vi "Initialize Steps Tree.vi"(11 "UI Data in":refnum<class "Settings UI.lvclass">) -> (2 "Items to Add":T1(array[cluster]), 3 "UI Data out":refnum<class "Settings UI.lvclass">)   [LabVIEW 2020, in "Output Sequencer.lvlib" / "Settings UI.lvclass"]
uses:
  Settings UI.lvclass
  Types/Tree Index Enum.ctl
  Settings UI.lvclass/Settings UI.ctl
  Globals/Global Tree Data.vi
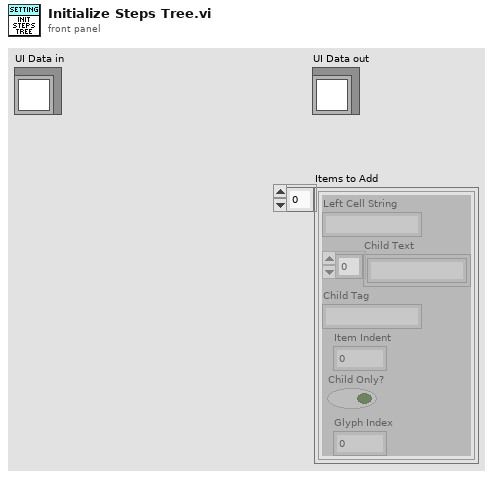
[diagram p1: front panel]
types:
  T1 = cluster{"Left Cell String":string, "Child Text":string[], "Child Tag":string, "Item Indent":i32, "Child Only?":bool, "Glyph Index":i32}[]
  T2 = typedef "Output Sequencer.lvlib/Settings UI.lvclass/Tree Index Enum.ctl" = enum16{"General Settings", "Num Steps", "Num Analog", "Num Digital", "Show Confirmation", "Interp Priority", "Adv Timing", "Enable Conditions", "Seq Execution", "Reset Test Start", "Only When Test", "Delay After Test", "Start condition", "Re-triggering", "Stop condition", "Stop After Cycles", "Stop Values", "Default Values", "Default Analog", "Default Digital", "Steps", "Step #", "Description", "Precondition", "Duration", "Mode", "Delay Between Vals", "Analog Values", "Digital Values", "Postcondition", "On True", "On False"}
  T3 = typedef "Output Sequencer.lvlib/Settings UI.lvclass/Step Settings.ctl" = cluster{"Description":string, "Precondition":string, "Duration":dbl, "Mode":string, "Delay Between Values":dbl, "Analog Values":string[], "Digital Values":string[], "Postcondition":string, "On True":string, "On False":string}
  T4 = cluster{"Left Cell String":string, "Child Text":string[], "Child Tag":string, "Item Indent":i32, "Child Only?":bool, "Glyph Index":i32}
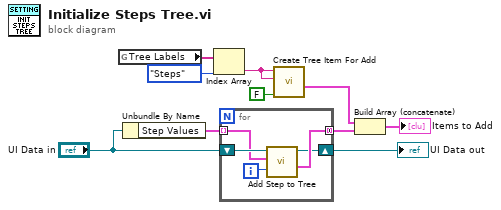
[diagram p0: block diagram]
diagram:
  n1 = global read "Global Tree Data.vi" "Tree Labels"() -> (w7:string[])
  n2 = Unbundle By Name("UI Data in") -> ("Step Values"=w8:T3[])
  n3 = Index Array(array=w7, index=Tree_Index_Enum."Steps" ("Tree Index Enum")) -> (element=w6:string)
  n4 = for {
    tunnel: w8 -> [w11] mode=indexing
    tunnel: [w14] -> w3 mode=concatenating
    shift-right: [w12] -> w1
    shift-left: "UI Data in" -> [w13]
    i -> [w15]
    n5 = call "Add Step to Tree.vi"("Step Index"=w15, "Step Settings"=w11, "UI Data In"=w13) -> ("Tree Items"=w14:T1, "UI Data out"=w12:refnum<class "Settings UI.lvclass">)  [unwired: 6 in, 1 out]
  }
  "UI Data out" <- w1
  n6 = call "Create Tree Item For Add.vi"("Child Only? (true)"=FALSE, "Left Cell String"=w6, "Child Tag in"=w6) -> ("Item"=w2:T4)  [unwired: 7 in, 1 out]
  n7 = Build Array (concatenate)(w2, w3) -> (→"Items to Add":T1)
